vi "CSV_Query.vi"(0 "System no.":i32=1 min=1 max=4 step=1, 5 "error in":errorcluster) -> (14 "Syntax":T1=enum."GCS 2.0", 19 "error out":errorcluster)   [LabVIEW 2020]
doc: "GCS 3.0\n=====\n\nCSV? (Get GCS Version)\n\nDescription \nQueries the GCS syntax version used in the firmware.\n\nFormat\nCSV?\n\nArguments\nnone\n\nResponse\n3.0\n\nExample\n>>CSV?\n<<3.0\n\nNotes\nSoftware from PI, such as PIMikroMove, uses the response to CSV? to adapt to the GCS version \nof the connected controller. GCS 2.0 and 3.0 differ, for example, in the access to the data \nrecorder.\n\nUser command level\nUSR\n\n\nGCS 2.0\n=====\n\nReturns current GCS syntax version. \n\nC-887, F-206, M-8X0: Only for GCS syntax version = GCS 2.0 or higher (check with CSV?.vi. If CSV?.vi is not supported, syntax version is GCS 1.0)."
uses:
  Syntax.ctl
panel:
  # "CSV? (Get GCS Version)\n\nQueries the GCS syntax version used in the firmware."
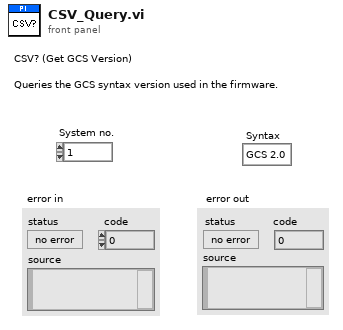
[diagram p1: front panel]
types:
  T1 = typedef "Syntax.ctl" = enum16{"GCS 1.0", "GCS 2.0", "GCS 3.0"}
  T2 = enum16{"Disable error check", "Force error check", "Use global settings"}
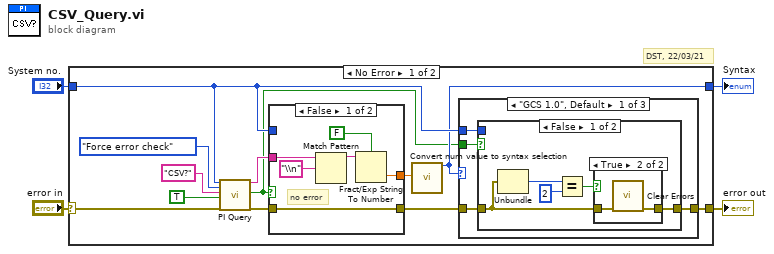
[diagram p0: block diagram]
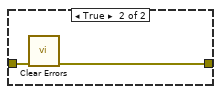
[diagram p3: hidden frame]
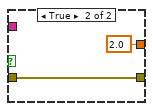
[diagram p6: hidden frame]
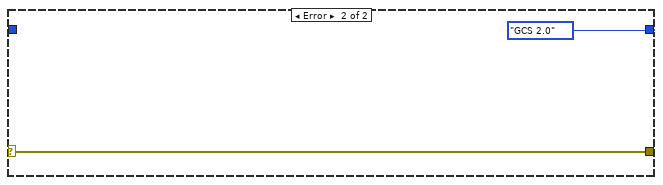
[diagram p7: hidden frame]
diagram:
  # "DST, 22/03/21"
  n1 = case shown="No Error" "error in" {
    selector: "error in" -> [w9 w42]
    tunnel: [w14 w42] -> w4
    tunnel: "System no." -> [w11 _]
    tunnel: [w6 Syntax."GCS 2.0" ("Syntax")] -> w1
    frame No Error {
      n2 = call "PI Query.vi"("System no."=w11, "Error check settings"=T2."Force error check", "String to send"="CSV?", "Attach termination char.?"=TRUE ("Attach Linefeed?"), "error in"=w9) -> ("String read"=w10:string, "Controller error"=w5:bool, "error out"=w7:errorcluster)  [unwired: 2 in, 10 out]
      n3 = case shown="False" w5 {
        tunnel: w10 -> [w38 _]
        tunnel: [w35 2.0] -> w16
        tunnel: w11 -> [_ _]
        tunnel: w7 -> [w33 w39]
        tunnel: [w33 w39] -> w15
        frame False {
          # "no error"
          n4 = Match Pattern(string=w38, regular expression="\\n") -> (before substring=w36:string)  [unwired: 4 out]
          n5 = Fract/Exp String To Number(use system decimal point (T)=FALSE, string=w36) -> (number=w35:dbl)  [unwired: 3 out]
        }
        frame True {
        }
      }
      n6 = call "Convert num value to syntax selection.vi"("GCS syntax version"=w16) -> ("Syntax"=w6:T1)  [unwired: 18 out]
      n7 = case shown="\"GCS 1.0\", Default" w6 {
        tunnel: w15 -> [w20 w31 w32]
        tunnel: [w17 w31 w32] -> w14
        tunnel: w11 -> [w19 _ _]
        tunnel: w5 -> [w18 _ _]
        frame "GCS 1.0", Default {
          n8 = case shown="False" w18 {
            tunnel: w20 -> [w21 w30]
            tunnel: w19 -> [_ _]
            tunnel: [w22 w29] -> w17
            frame False {
              n9 = Unbundle(w21) -> ("code"=w25:i32)  [unwired: 2 out]
              n10 = Equal?(x=w25, y=2) -> (x = y?=w23:bool)
              n11 = case shown="True" w23 {
                tunnel: [w26 w27] -> w22
                tunnel: w21 -> [w26 w28]
                frame False {
                }
                frame True {
                  n12 = call "Clear Errors.vi"("error in (no error)"=w28) -> ("error out"=w27:errorcluster)  [unwired: 1 in, 5 out]
                }
              }
            }
            frame True {
              n13 = call "Clear Errors.vi"("error in (no error)"=w30) -> ("error out"=w29:errorcluster)  [unwired: 1 in, 5 out]
            }
          }
        }
        frame "GCS 2.0" {
        }
        frame "GCS 3.0" {
        }
      }
    }
    frame Error {
    }
  }
  "error out" <- w4
  "Syntax" <- w1
